vi "FPGA Main.vi"() -> ()   [LabVIEW 2018]
doc: "This VI reads all analogue data channels available at the fastest rate supported by the respective hardware and updates a memory address for when each measurement is available.\n\nAt a rate defined by the fastest module (NI 9237 - default of 12.5kHz) this memory is read, combined with the measurements from the 9237 module and written to the FIFO for communication to the RT machine.\n\nThe NI 9237 modeul therefore defines the nominal sampling rate of the system (with slower channels over-sampled).\n\nA time channel (in uSec) is provided with 0 referenced from the first acquisition of the NI 9237 module"
uses:
  <vilib>/LabVIEW Targets/FPGA/cRIO/shared/nicrio_ModuleControls/nicrio_cRIO-9237_DataRatesRing.ctl
  <vilib>/Platform/TimedLoop/XDataNode/timing_clust.ctl
  <vilib>/Platform/TimedLoop/XDataNode/nitl_modes.ctl
  <vilib>/Platform/TimedLoop/XDataNode/wakeup.ctl
  <vilib>/rvi/Emulation/niFpgaGetClockAttributes.vi
  <vilib>/rvi/Emulation/niFpgaSctlEmulationGetInTimedLoop.vi
  <vilib>/rvi/Emulation/niFpgaEmulationReportErrorSimple.vi
  <vilib>/rvi/Emulation/niFpgaProcessEmulError.vi
  <vilib>/rvi/eio/common/nirviEmuTemplatePropertySet_noerrors.vi
  <vilib>/rvi/eio/common/nirviEmuTemplateMethod_errors.vi
  <vilib>/rvi/interface/RandomDataEmulation/niFpgaRandomDataHandleErrors.vi
  <vilib>/rvi/Memory/Memory_Emulation/nirvimemoryFastEmulation.vi
  <vilib>/rvi/Memory/Memory_Emulation/nirvimemoryEmulation.vi
  <vilib>/rvi/Emulation/niFpgaEmulationIsFPGAContextNoSignature.vi
  <vilib>/rvi/DataTransferAndStorage/Container/Common/niFpgaContainerGetUniqueNameForEmu.vi
  <vilib>/rvi/errors/nirviReportUnexpectedCaseInternalError (U32).vi
  <vilib>/rvi/Emulation/niFpgaCriticalErrorInLSC.vi
  <vilib>/eio/EIOPropertyNode/EIOPropertyNode.xnode
  <vilib>/eio/EIONode/EIONode.xnode
  <vilib>/rvi/DataTransferAndStorage/Container/XNode/niFpgaContainer.xnode
  <vilib>/rvi/interface/RandomDataEmulation/nirviRandomDataFpgaReadWriteTemplate.vi
  <vilib>/platform/TimedLoop/XDataNode/XDataNode.xnode
  <vilib>/eio/EIOMethodNode/EIOMethodNode.xnode
  <vilib>/Platform/TimedLoop/XDataNode/XDNodeRunTimeDep.lvlib
  <vilib>/rvi/eio/common/nirviEmuTemplatePropertyGet_errors.vi
  <vilib>/rvi/eio/common/nirviEmuTemplatePropertyGet_noerrors.vi
  <vilib>/rvi/eio/common/nirviEmuTemplatePropertySet_errors.vi
panel:
  in  "falling edge (F)":bool caption="Torque encoder direction"
  in  "filterTorque":bool
  in  "Data Rate":T1=1 items=["50.000 kS/s (NI 9237)"=1, "25.000 kS/s (NI 9237)"=2, "16.667 kS/s (NI 9237)"=3, "12.500 kS/s (NI 9237)"=4, "10.000 kS/s (NI 9237)"=5, "8.333 kS/s (NI 9237)"=6, "7.143 kS/s (NI 9237)"=7, "6.250 kS/s (NI 9237)"=8, "5.556 kS/s (NI 9237)"=9, "5.000 kS/s (NI 9237)"=10, "4.545 kS/s (NI 9237)"=11, "4.167 kS/s (NI 9237)"=12, "3.846 kS/s (NI 9237)"=13, "3.571 kS/s (NI 9237)"=14, "3.333 kS/s (NI 9237)"=15, "3.125 kS/s (NI 9237)"=16, "2.941 kS/s (NI 9237)"=17, "2.778 kS/s (NI 9237)"=18, "2.632 kS/s (NI 9237)"=19, "2.500 kS/s (NI 9237)"=20, "2.381 kS/s (NI 9237)"=21, "2.273 kS/s (NI 9237)"=22, "2.174 kS/s (NI 9237)"=23, "2.083 kS/s (NI 9237)"=24, "2.000 kS/s (NI 9237)"=25, "1.923 kS/s (NI 9237)"=26, "1.852 kS/s (NI 9237)"=27, "1.786 kS/s (NI 9237)"=28, "1.724 kS/s (NI 9237)"=29, "1.667 kS/s (NI 9237)"=30, "1.613 kS/s (NI 9237)"=31]
  in  "encoders offset":sgl caption="encoder offset (radians)"
  out "Total channel count":u32=61
  out "timestamp":u32
  out "FIFO full counter":i32
  in  "Safe Voltage":fxp<+/-,20,5>[](array[numeric])=[0.0, 0.0, 0.0, 0.0]
  in  "Safe Digital":bool[](array[boolean])=[FALSE, FALSE, FALSE, FALSE, FALSE, FALSE, FALSE, FALSE]
  in  "Voltage Out":fxp<+/-,20,5>[](array[numeric])=[0.0, 0.0, 0.0, 0.0]
  in  "Update Outputs":bool
  in  "Mod 8":bool[](array[boolean])=[FALSE, FALSE, FALSE, FALSE, FALSE, FALSE, FALSE, FALSE]
  out "E Stop":bool
  in  "Stop acquire":bool
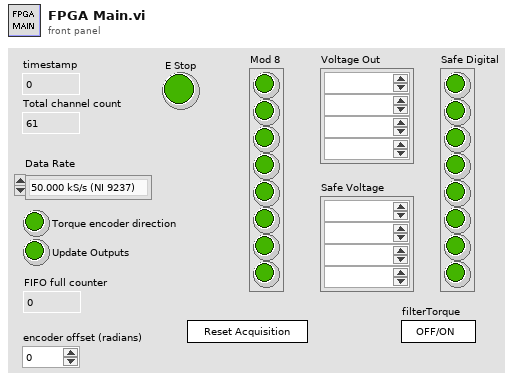
[diagram p1: front panel]
types:
  T1 = typedef "nicrio_cRIO-9237_DataRatesRing.ctl" = u8
  T2 = typedef "XDNodeRunTimeDep.lvlib/timing_clust.ctl" = cluster{"Expected End [f-1]":u64, "Actual End [f-1]":u64, "Finished Late? [f-1]":bool, "Expected End [i-1]":u64, "Actual End [i-1]":u64, "Finished Late? [i-1]":bool, "Expected Start [i]":u64, "Actual Start [i]":u64, "Expected Start [f]":u64, "Actual Start [f]":u64, "Source Name":string, "Structure Name":string, "Period":i64, "Deadline":i64, "Offset":i64, "Start":i64, "Priority":i32, "Timeout":i32, "Mode":T3, "Wakeup Reason":T4, "Error":errorcluster, "Source Type":string, "Secondary Source Type":string, "Global End Time":u64, "Global Start Time":u64, "Frame Duration":u64, "Iteration Duration":u64, "Assigned CPU":i32, "I/O Scan Engine Mode":u32}
  T3 = typedef "XDNodeRunTimeDep.lvlib/nitl_modes.ctl" = enum32{"No Change", "Process missed periods, maintain original phase", "Discard missed periods, maintain original phase", "Process missed periods, ignore original phase", "Discard missed periods, ignore original phase"}
  T4 = typedef "XDNodeRunTimeDep.lvlib/wakeup.ctl" = enum32{"Normal", "Aborted", "Asynchronous wakeup", "Timing source error", "Timed loop error", "Timeout"}
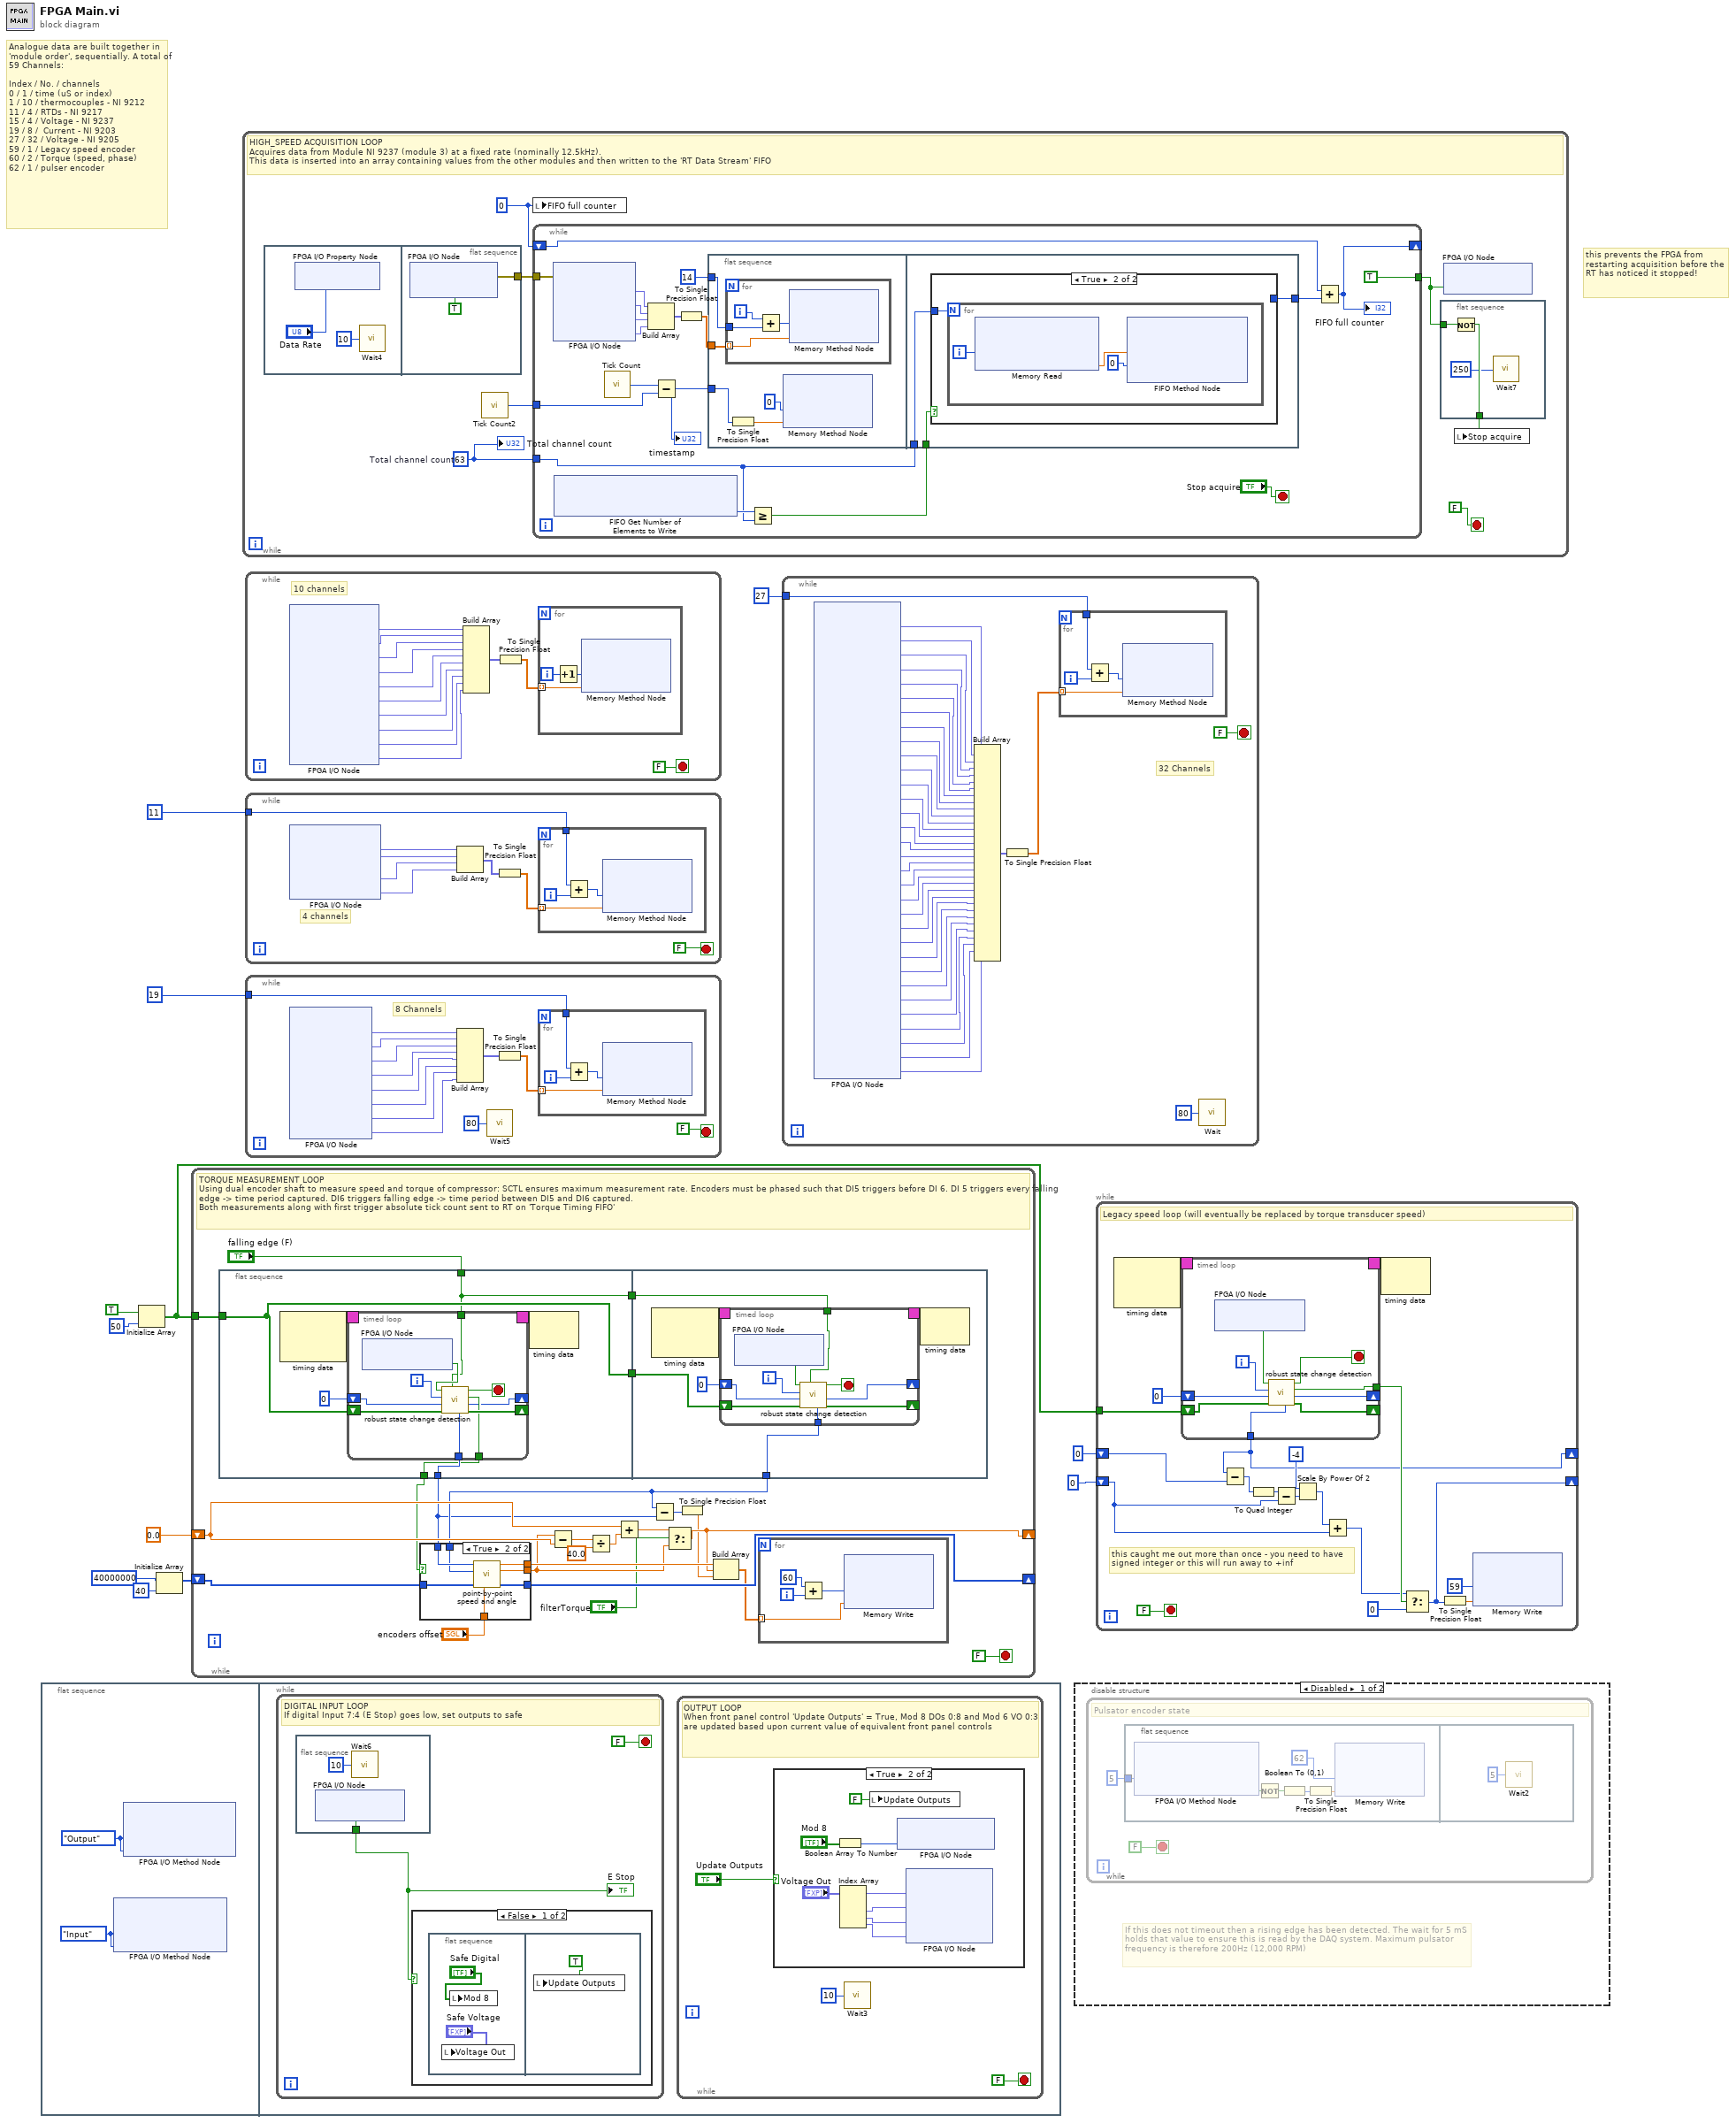
[diagram p0: block diagram]
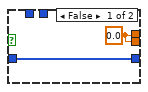
[diagram p5: hidden frame]
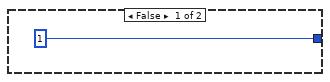
[diagram p6: hidden frame]
diagram:
  # "this prevents the FPGA from restarting acquisition before the RT has noticed it stopped!"
  # "Analogue data are built together in 'module order', sequentially. A total of 59 Channels:\n\nIndex / No. / channels\n0 / 1 / time (uS or index)\n1 / 10 / thermocouples - NI 9212\n11 / 4 / RTDs - NI 9217\n15 / 4 / Voltage - NI 9237\n19 / 8 /  Current - NI 9203\n27 / 32 / Voltage - NI 9205\n59 / 1 / Legacy speed encoder\n60 / 2 / Torque (speed, phase)\n62 / 1 / pulser encoder"
  n1 = flat-sequence {
    frame #0 {
      w13 = enum8{"No Change", "Input", "Output"}."Output" ("DIO 7:4")
      w14 = enum8{"No Change", "Input", "Output"}."Input" ("DIO 7:4")
      n2 = xnode "FPGA I/O Method Node"("DIO 7:4"=w14, "DIO 3:0"=w14) -> ()  [unwired: 1 in, 1 out]
      n3 = xnode "FPGA I/O Method Node"("DIO 7:4"=w13, "DIO 3:0"=w13) -> ()  [unwired: 1 in, 1 out]
    }
    frame #1 {
      n4 = while {
        stop <- FALSE stop-if-true
        # "DIGITAL INPUT LOOP\nIf digital Input 7:4 (E Stop) goes low, set outputs to safe"
        n5 = flat-sequence {
          tunnel: [w29] -> w26
          frame #0 {
            n6 = xnode "FPGA I/O Node"() -> ("Mod7/DIO4"=w29:bool)  [unwired: 1 in, 1 out]
            n7 = call "Wait6"("Count(uSec)"=u8 10) -> ()  [unwired: 1 out]
          }
        }
        n8 = case shown="False" w26 {
          frame False {
            n9 = flat-sequence {
              frame #0 {
                n10 = local write "Voltage Out"("Safe Voltage") -> ()
                n11 = local write "Mod 8"("Safe Digital") -> ()
              }
              frame #1 {
                n12 = local write "Update Outputs"(TRUE ("Update Outputs")) -> ()
              }
            }
          }
          frame True {
          }
        }
        "E Stop" <- w26
      }
      n13 = while {
        stop <- FALSE stop-if-true
        # "OUTPUT LOOP\nWhen front panel control 'Update Outputs' = True, Mod 8 DOs 0:8 and Mod 6 VO 0:3 are updated based upon current value of equivalent front panel controls"
        n14 = case shown="True" "Update Outputs" {
          frame False {
          }
          frame True {
            n15 = Boolean Array To Number(Boolean array="Mod 8") -> (number=w24:u8)
            n16 = Index Array(array="Voltage Out") -> (element #1=w22:fxp<+/-,20,5>, element #2=w21:fxp<+/-,20,5>, element #3=w20:fxp<+/-,20,5>, element #4=w19:fxp<+/-,20,5>)  [unwired: 4 in]
            n17 = local write "Update Outputs"(FALSE ("Update Outputs")) -> ()
            n18 = xnode "FPGA I/O Node"("Mod8/DIO7:0"=w24) -> ()  [unwired: 1 in, 1 out]
            n19 = xnode "FPGA I/O Node"("Mod6/AO0"=w22, "Mod6/AO1"=w21, "Mod6/AO2"=w20, "Mod6/AO3"=w19) -> ()  [unwired: 4 in, 4 out]
          }
        }
        n20 = call "Wait3"("Count(uSec)"=u16 10 ("Count(Ticks)")) -> ()  [unwired: 1 out]
      }
    }
  }
  n21 = Initialize Array(TRUE, 50 ("edge buffer size")) -> (w2:bool[])
  n22 = Initialize Array(u32 40000000 ("64bit integer"), 40 ("dimension size")) -> (w7:u32[])
  n23 = while {
    shift-right: [w53] -> _
    shift-left: w7 -> [w54]
    shift-right: [w40] -> _
    shift-left: sgl 0.0 -> [w49]
    tunnel: w2 -> [w47]
    stop <- FALSE stop-if-true
    # "TORQUE MEASUREMENT LOOP\nUsing dual encoder shaft to measure speed and torque of compressor: SCTL ensures maximum measurement rate. Encoders must be phased such that DI5 triggers before DI 6. DI 5 triggers every falling edge -> time period captured. DI6 triggers falling edge -> time period between DI5 and DI6 captured.\nBoth measurements along with first trigger absolute tick count sent to RT on 'Torque Timing FIFO'"
    n24 = flat-sequence {
      tunnel: [w73] -> w35
      tunnel: [w72] -> w48
      tunnel: w47 -> [w70]
      tunnel: [w70] -> w46
      tunnel: "falling edge (F)" -> [w69]
      tunnel: [w69] -> w33
      tunnel: [w95] -> w36
      tunnel: w46 -> [w94]
      tunnel: w33 -> [w90]
      frame #0 {
        n25 = node-c288() -> (w75:T2)  [unwired: 2 in]
        n26 = timed-loop {
          timing: w75 -> [_]
          timing-out: [_] -> w74
          tunnel: [w80] -> w73
          tunnel: [w79] -> w72
          shift-right: [w83] -> _
          shift-left: w70 -> [w84]
          shift-right: [w77] -> _
          shift-left: i16 0 ("step") -> [w81]
          tunnel: w69 -> [w76]
          i -> [w82]
          stop <- w78 stop-if-true
          n27 = xnode "FPGA I/O Node"() -> ("Mod7/DIO0"=w85:bool)  [unwired: 1 in, 1 out]
          n28 = call "robust state change detection.vi"("falling edge (F)"=w76, "history"=w84, "step"=w81, "tick"=w82, "New state"=w85) -> ("history out"=w83:bool[], "step out"=w77:i16, "edge detected"=w79:bool, "Stop?"=w78:bool, "tick"=w80:u32)  [unwired: 2 in]
        }
        n29 = node-c288(w74) -> ()  [unwired: 1 out]
      }
      frame #1 {
        n30 = node-c288() -> (w93:T2)  [unwired: 2 in]
        n31 = timed-loop {
          timing: w93 -> [_]
          timing-out: [_] -> w92
          shift-right: [w102] -> _
          shift-left: w94 -> [w103]
          tunnel: [w100] -> w95
          shift-right: [w97] -> _
          shift-left: i16 0 ("step") -> [w98]
          tunnel: w90 -> [w96]
          i -> [w99]
          stop <- w101 stop-if-true
          n32 = xnode "FPGA I/O Node"() -> ("Mod7/DIO1"=w104:bool)  [unwired: 1 in, 1 out]
          n33 = call "robust state change detection.vi"("falling edge (F)"=w96, "history"=w103, "step"=w98, "tick"=w99, "New state"=w104) -> ("history out"=w102:bool[], "step out"=w97:i16, "Stop?"=w101:bool, "tick"=w100:u32)  [unwired: 2 in, 1 out]
        }
        n34 = node-c288(w92) -> ()  [unwired: 1 out]
      }
    }
    n35 = case shown="True" w48 {
      tunnel: w35 -> [_ w64]
      tunnel: w36 -> [_ w63]
      tunnel: w54 -> [w57 w62]
      tunnel: [w57 w61] -> w53
      tunnel: "encoders offset" -> [_ w58]
      tunnel: [w56 w60] -> w51
      tunnel: [w56 w59] -> w41
      frame False {
        w56 = sgl 0.0 ("calculated speed (Hz)")
      }
      frame True {
        n36 = call "point-by-point speed and angle.vi"("encoder fixed offest"=w58, "speed history in"=w62, "angle pulse"=w63, "speed pulse"=w64) -> ("speed history out"=w61:u32[], "calculated angle (radians)"=w59:sgl, "calculated speed (rad/tick)"=w60:sgl)  [unwired: 5 in]
      }
    }
    n37 = Subtract(x=w41, y=w49) -> (x-y=w45:sgl)
    n38 = Divide(x=w45, y=sgl 40.0) -> (x/y=w43:sgl)
    n39 = Add(x=w49, y=w43) -> (x+y=w42:sgl)
    n40 = Subtract(x=w36, y=w35) -> (x-y=w37:u32)
    n41 = Select(t=w42, s="filterTorque", f=w41) -> (s? t:f=w40:sgl)
    n42 = To Single Precision Float(number=w37) -> (single precision float=w38:sgl)
    n43 = Build Array(w51, w40, w38) -> (w50:sgl[])
    n44 = for {
      tunnel: w50 -> [w65] mode=indexing
      i -> [w66]
      n45 = Add(x=u32 60 ("Address"), y=w66) -> (x+y=w67:u32)
      n46 = xnode ("Memory Write")("Address"=w67, "Data"=w65) -> ()  [unwired: 1 in, 1 out]
    }
  }
  n47 = while {
    stop <- FALSE stop-if-true
    w110 = 0 ("FIFO full counter")
    w113 = u32 63  # Total channel count
    # "HIGH_SPEED ACQUISITION LOOP\nAcquires data from Module NI 9237 (module 3) at a fixed rate (nominally 12.5kHz).\nThis data is inserted into an array containing values from the other modules and then written to the 'RT Data Stream' FIFO"
    n48 = flat-sequence {
      tunnel: [w122] -> w114
      frame #0 {
        n49 = xnode "FPGA I/O Property Node"("Data Rate"="Data Rate") -> ()  [unwired: 1 in, 1 out]
        n50 = call "Wait4"("Count(mSec)"=u16 10) -> ()  [unwired: 1 out]
      }
      frame #1 {
        n51 = xnode "FPGA I/O Node"("Mod3/Start"=TRUE) -> ("error out"=w122:errorcluster)  [unwired: 2 in, 1 out]
      }
    }
    n52 = call "Tick Count2"() -> ("Tick Count(uSec)"=w115:u32)
    n53 = local write "FIFO full counter"(w110) -> ()
    n54 = while {
      tunnel: [TRUE ("I/O Item")] -> w112
      tunnel: w114 -> [w140]
      tunnel: w113 -> [w125]
      shift-right: [w133] -> _
      shift-left: w110 -> [w131]
      tunnel: w115 -> [w134]
      stop <- "Stop acquire" stop-if-true
      n55 = xnode "FPGA I/O Node"("error in"=w140) -> ("Mod3/AI0"=w139:fxp<+/-,24,-4>, "Mod3/AI1"=w138:fxp<+/-,24,-4>, "Mod3/AI2"=w137:fxp<+/-,24,-4>, "Mod3/AI3"=w136:fxp<+/-,24,-4>)  [unwired: 4 in, 5 out]
      n56 = xnode ("FIFO Get Number of Elements to Write")() -> ("Number of Elements to Write"=w127:u32)  [unwired: 1 in, 1 out]
      n57 = call "Tick Count"() -> ("Tick Count(uSec)"=w130:u32)
      n58 = Build Array(w139, w138, w137, w136) -> (w135:fxp<+/-,24,-4>[])
      n59 = Subtract(x=w130, y=w134) -> (x-y=w123:u32)
      "timestamp" <- w123
      n60 = To Single Precision Float(number=w135) -> (single precision float=w129:sgl[])
      n61 = flat-sequence {
        tunnel: w129 -> [w146]
        tunnel: 14 ("index") -> [w145]
        tunnel: w123 -> [w143]
        tunnel: w125 -> [w153]
        tunnel: [w152] -> w124
        tunnel: w126 -> [w151]
        frame #0 {
          n62 = for {
            tunnel: w146 -> [w150] mode=indexing
            tunnel: w145 -> [w149]
            i -> [w147]
            n63 = Add(x=w147, y=w149) -> (x+y=w148:i32)
            n64 = xnode ("Memory Method Node")("Address"=w148, "Data"=w150) -> ()  [unwired: 1 in, 1 out]
          }
          n65 = To Single Precision Float(number=w143) -> (single precision float=w144:sgl)
          n66 = xnode ("Memory Method Node")("Address"=u32 0, "Data"=w144) -> ()  [unwired: 1 in, 1 out]
        }
        frame #1 {
          n67 = case shown="True" w151 {
            tunnel: [1 _] -> w152
            tunnel: w153 -> [_ w155]
            frame False {
            }
            frame True {
              n68 = for {
                N: w155 -> [_]
                i -> [w156]
                n69 = xnode ("Memory Read")("Address"=w156) -> ("Data"=w157:sgl)  [unwired: 1 in, 1 out]
                n70 = xnode ("FIFO Method Node")("Element"=w157, "Timeout"=0) -> ()  [unwired: 1 in, 2 out]
              }
            }
          }
        }
      }
      n71 = Greater Or Equal?(x=w127, y=w125) -> (x >= y?=w126:bool)
      n72 = Add(x=w131, y=w124) -> (x+y=w133:i32)
      "FIFO full counter" <- w133
    }
    n73 = flat-sequence {
      tunnel: w112 -> [w118]
      tunnel: [w117] -> w109
      frame #0 {
        n74 = Not(x=w118) -> (.not. x?=w117:bool)
        n75 = call "Wait7"("Count(mSec)"=u8 250) -> ()  [unwired: 1 out]
      }
    }
    n76 = xnode "FPGA I/O Node"("Mod3/Stop"=w112) -> ()  [unwired: 1 in, 1 out]
    n77 = local write "Stop acquire"(w109) -> ()
    "Total channel count" <- w113
  }
  n78 = while {
    stop <- FALSE stop-if-true
    # "10 channels"
    n79 = xnode "FPGA I/O Node"() -> ("Mod1/TC0"=w171:fxp<+/-,24,-2>, "Mod1/TC1"=w170:fxp<+/-,24,-2>, "Mod1/TC2"=w169:fxp<+/-,24,-2>, "Mod1/TC3"=w168:fxp<+/-,24,-2>, "Mod1/TC4"=w167:fxp<+/-,24,-2>, "Mod1/TC5"=w166:fxp<+/-,24,-2>, "Mod1/TC6"=w165:fxp<+/-,24,-2>, "Mod1/TC7"=w164:fxp<+/-,24,-2>, "Mod1/CJC0"=w161:fxp<+/-,24,-2>, "Mod1/CJC1"=w160:fxp<+/-,24,-2>)  [unwired: 10 in, 10 out]
    n80 = Build Array(w171, w170, w169, w168, w167, w166, w165, w164, w161, w160) -> (w163:fxp<+/-,24,-2>[])
    n81 = To Single Precision Float(number=w163) -> (single precision float=w162:sgl[])
    n82 = for {
      tunnel: w162 -> [w174] mode=indexing
      i -> [w173]
      n83 = Increment(x=w173) -> (x+1=w172:i32)
      n84 = xnode ("Memory Method Node")("Address"=w172, "Data"=w174) -> ()  [unwired: 1 in, 1 out]
    }
  }
  n85 = while {
    tunnel: 11 ("Numeric") -> [w176]
    stop <- FALSE stop-if-true
    # "4 channels"
    n86 = xnode "FPGA I/O Node"() -> ("Mod2/RTD0"=w182:fxp<+/-,24,10>, "Mod2/RTD1"=w181:fxp<+/-,24,10>, "Mod2/RTD2"=w180:fxp<+/-,24,10>, "Mod2/RTD3"=w177:fxp<+/-,24,10>)  [unwired: 4 in, 4 out]
    n87 = Build Array(w182, w181, w180, w177) -> (w179:fxp<+/-,24,10>[])
    n88 = To Single Precision Float(number=w179) -> (single precision float=w178:sgl[])
    n89 = for {
      tunnel: w178 -> [w186] mode=indexing
      tunnel: w176 -> [w183]
      i -> [w185]
      n90 = Add(x=w183, y=w185) -> (x+y=w184:i32)
      n91 = xnode ("Memory Method Node")("Address"=w184, "Data"=w186) -> ()  [unwired: 1 in, 1 out]
    }
  }
  n92 = while {
    tunnel: 19 ("Numeric") -> [w193]
    stop <- FALSE stop-if-true
    # "8 Channels"
    n93 = xnode "FPGA I/O Node"() -> ("Mod4/AI0"=w199:fxp<+/-,21,-4>, "Mod4/AI1"=w198:fxp<+/-,21,-4>, "Mod4/AI2"=w197:fxp<+/-,21,-4>, "Mod4/AI3"=w194:fxp<+/-,21,-4>, "Mod4/AI4"=w192:fxp<+/-,21,-4>, "Mod4/AI5"=w191:fxp<+/-,21,-4>, "Mod4/AI6"=w190:fxp<+/-,21,-4>, "Mod4/AI7"=w189:fxp<+/-,21,-4>)  [unwired: 8 in, 8 out]
    n94 = Build Array(w199, w198, w197, w194, w192, w191, w190, w189) -> (w196:fxp<+/-,21,-4>[])
    n95 = call "Wait5"("Count(uSec)"=u8 80) -> ()  [unwired: 1 out]
    n96 = To Single Precision Float(number=w196) -> (single precision float=w195:sgl[])
    n97 = for {
      tunnel: w195 -> [w203] mode=indexing
      tunnel: w193 -> [w200]
      i -> [w202]
      n98 = Add(x=w200, y=w202) -> (x+y=w201:i32)
      n99 = xnode ("Memory Method Node")("Address"=w201, "Data"=w203) -> ()  [unwired: 1 in, 1 out]
    }
  }
  n100 = while {
    tunnel: 27 ("Numeric") -> [w239]
    stop <- FALSE stop-if-true
    # "32 Channels"
    n101 = xnode "FPGA I/O Node"() -> ("Mod5/AI0"=w207:fxp<+/-,26,5>, "Mod5/AI1"=w208:fxp<+/-,26,5>, "Mod5/AI2"=w209:fxp<+/-,26,5>, "Mod5/AI3"=w210:fxp<+/-,26,5>, "Mod5/AI4"=w211:fxp<+/-,26,5>, "Mod5/AI5"=w212:fxp<+/-,26,5>, "Mod5/AI6"=w213:fxp<+/-,26,5>, "Mod5/AI7"=w214:fxp<+/-,26,5>, "Mod5/AI8"=w238:fxp<+/-,26,5>, "Mod5/AI9"=w237:fxp<+/-,26,5>, "Mod5/AI10"=w236:fxp<+/-,26,5>, "Mod5/AI11"=w235:fxp<+/-,26,5>, "Mod5/AI12"=w234:fxp<+/-,26,5>, "Mod5/AI13"=w233:fxp<+/-,26,5>, "Mod5/AI14"=w232:fxp<+/-,26,5>, "Mod5/AI15"=w231:fxp<+/-,26,5>, "Mod5/AI16"=w230:fxp<+/-,26,5>, "Mod5/AI17"=w229:fxp<+/-,26,5>, "Mod5/AI18"=w228:fxp<+/-,26,5>, "Mod5/AI19"=w227:fxp<+/-,26,5>, "Mod5/AI20"=w226:fxp<+/-,26,5>, "Mod5/AI21"=w225:fxp<+/-,26,5>, "Mod5/AI22"=w224:fxp<+/-,26,5>, "Mod5/AI23"=w223:fxp<+/-,26,5>, "Mod5/AI24"=w222:fxp<+/-,26,5>, "Mod5/AI25"=w221:fxp<+/-,26,5>, "Mod5/AI26"=w220:fxp<+/-,26,5>, "Mod5/AI27"=w219:fxp<+/-,26,5>, "Mod5/AI28"=w218:fxp<+/-,26,5>, "Mod5/AI29"=w217:fxp<+/-,26,5>, "Mod5/AI30"=w216:fxp<+/-,26,5>, "Mod5/AI31"=w215:fxp<+/-,26,5>)  [unwired: 32 in, 32 out]
    n102 = Build Array(w207, w208, w209, w210, w211, w212, w213, w214, w238, w237, w236, w235, w234, w233, w232, w231, w230, w229, w228, w227, w226, w225, w224, w223, w222, w221, w220, w219, w218, w217, w216, w215) -> (w240:fxp<+/-,26,5>[])
    n103 = To Single Precision Float(number=w240) -> (single precision float=w206:sgl[])
    n104 = for {
      tunnel: w206 -> [w244] mode=indexing
      tunnel: w239 -> [w241]
      i -> [w243]
      n105 = Add(x=w241, y=w243) -> (x+y=w242:i32)
      n106 = xnode ("Memory Method Node")("Address"=w242, "Data"=w244) -> ()  [unwired: 1 in, 1 out]
    }
    n107 = call "Wait"("Count(uSec)"=u8 80) -> ()  [unwired: 1 out]
  }
  n108 = disable-structure shown="Disabled" {
    frame Disabled {
      # "If this does not timeout then a rising edge has been detected. The wait for 5 mS holds that value to ensure this is read by the DAQ system. Maximum pulsator frequency is therefore 200Hz (12,000 RPM)"
      n109 = while {
        stop <- FALSE stop-if-true
        # "Pulsator encoder state"
        n110 = flat-sequence {
          tunnel: 5 ("Timeout") -> [w249]
          frame #0 {
            n111 = xnode "FPGA I/O Method Node"("Timeout"=w249) -> ("Timed Out"=w248:bool)  [unwired: 1 in, 1 out]
            n112 = Not(x=w248) -> (.not. x?=w247:bool)
            n113 = Boolean To (0,1)(Boolean=w247) -> (0, 1=w252:i16)
            n114 = To Single Precision Float(number=w252) -> (single precision float=w251:sgl)
            n115 = xnode ("Memory Write")("Address"=u32 62, "Data"=w251) -> ()  [unwired: 1 in, 1 out]
          }
          frame #1 {
            n116 = call "Wait2"("Count(mSec)"=u16 5 ("Count(uSec)")) -> ()  [unwired: 1 out]
          }
        }
      }
    }
    frame Enabled {
    }
  }
  n117 = while {
    shift-right: [w259] -> _
    shift-left: i64 0 -> [w266]
    tunnel: w2 -> [w260]
    shift-right: [w255] -> _
    shift-left: u32 0 ("tick") -> [w254]
    stop <- FALSE stop-if-true
    # "this caught me out more than once - you need to have signed integer or this will run away to +inf"
    # "Legacy speed loop (will eventually be replaced by torque transducer speed)"
    n118 = node-c288() -> (w272:T2)  [unwired: 2 in]
    n119 = timed-loop {
      timing: w272 -> [_]
      timing-out: [_] -> w271
      shift-right: [w278] -> _
      shift-left: i16 0 ("step") -> [w279]
      tunnel: [w276] -> w261
      tunnel: [w275] -> w255
      shift-right: [w273] -> _
      shift-left: w260 -> [w274]
      i -> [w280]
      stop <- w277 stop-if-true
      n120 = xnode "FPGA I/O Node"() -> ("Mod7/DIO3"=w281:bool)  [unwired: 1 in, 1 out]
      n121 = call "robust state change detection.vi"("history"=w274, "step"=w279, "tick"=w280, "New state"=w281) -> ("history out"=w273:bool[], "step out"=w278:i16, "edge detected"=w276:bool, "Stop?"=w277:bool, "tick"=w275:u32)  [unwired: 3 in]
    }
    n122 = Subtract(x=w255, y=w254) -> (x-y=w256:u32)
    n123 = To Quad Integer(1:w256) -> (0:w263:i64)
    n124 = Subtract(x=w263, y=w266) -> (x-y=w267:i64)
    n125 = Scale By Power Of 2(n=i16 -4, x=w267) -> (x*2^n=w269:i64)
    n126 = Add(x=w269, y=w266) -> (x+y=w257:i64)
    n127 = node-c288(w271) -> ()  [unwired: 1 out]
    n128 = Select(t=w257, s=w261, f=u32 0 ("t")) -> (s? t:f=w259:i64)
    n129 = To Single Precision Float(number=w259) -> (single precision float=w265:sgl)
    n130 = xnode ("Memory Write")("Address"=u32 59, "Data"=w265) -> ()  [unwired: 1 in, 1 out]
  }
